vi "WaitNextMultipleTime.vi"(10 "Error in":errorcluster, 11 "Wait Time":u32) -> (7 "Error out":errorcluster)   [LabVIEW 2016]
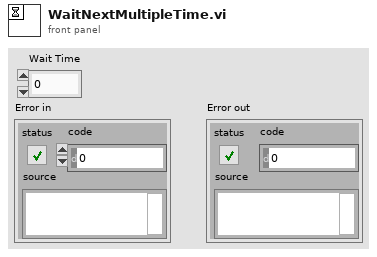
[diagram p1: front panel]
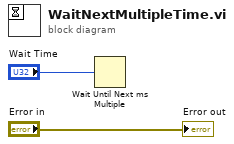
[diagram p0: block diagram]
diagram:
  n1 = Wait Until Next ms Multiple(millisecond multiple="Wait Time") -> ()  [unwired: 1 out]
  "Error out" <- "Error in"
